vi "xml_get_target.vi"(3 "error in (no error)":errorcluster, 4 "XML Path":path=path "D:/Test Management/Farmer/XML/targets.xml", 5 "target name":string) -> (0 "error out":errorcluster, 1 "success?":bool, 2 "Data":T1)   [LabVIEW 2011]
uses:
  TargetData.ctl
  <vilib>/xml/Load XML File.vi
  <vilib>/xml/Close Reference(Node).vi
  <vilib>/xml/NI_XML.lvlib
  Program Files/National Instruments/LabVIEW 2011/resource/objmgr/DOMUserDefRef.rc
panel:
  in  "data type":T1
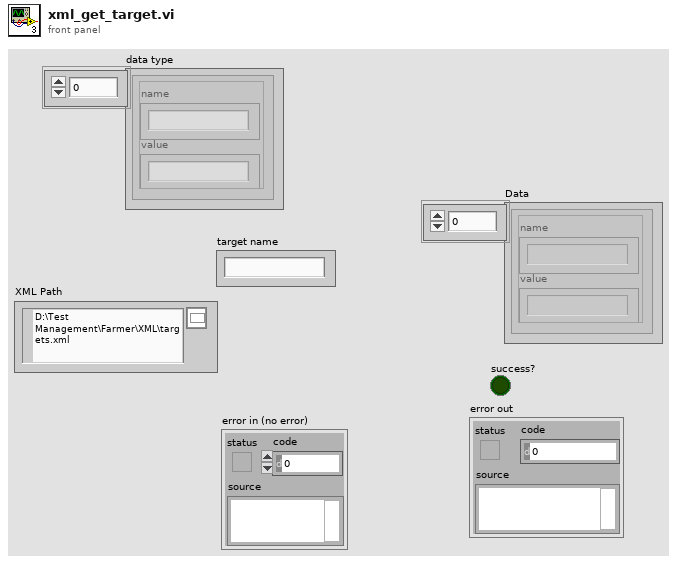
[diagram p1: front panel]
types:
  T1 = typedef "TargetData.ctl" = cluster{"name":string, "value":string}[]
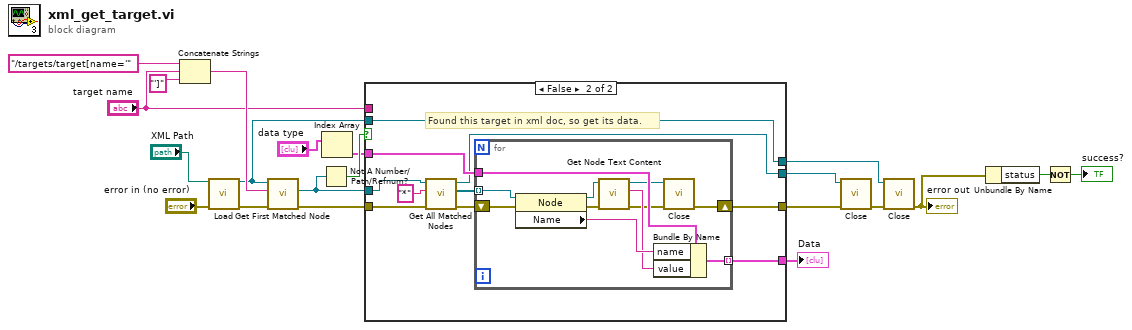
[diagram p0: block diagram]
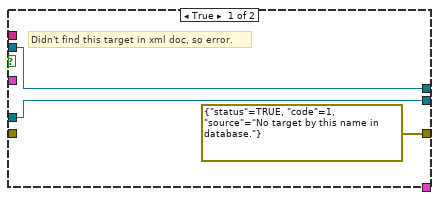
[diagram p2: hidden frame]
diagram:
  n1 = Concatenate Strings("/targets/target[name='", "target name", "']") -> (w19:string)
  n2 = call-poly <vilib>:"Load.vi"("path to XML document"="XML Path", "error in (no error)"="error in (no error)") -> ("DOM document out"=w6:refnum<k20>, "error out"=w18:errorcluster)  [unwired: 11 in, 1 out]
  n3 = call <vilib>:"Get First Matched Node.vi"("error in (no error)"=w18, "XPath expression"=w19, "node in"=w6) -> ("error out"=w17:errorcluster, "node result"=w14:refnum<k20>)  [unwired: 6 in, 1 out]
  n4 = Not A Number/Path/Refnum?(number/path/refnum=w14) -> (NaN/Path/Refnum?=w16:bool)
  n5 = Index Array(array="data type") -> (element=w3:cluster{"name":string, "value":string})  [unwired: 1 in]
  n6 = case shown="False" w16 {
    tunnel: w17 -> [_ w31]
    tunnel: [errorcluster {"status"=TRUE, "code"=1, "source"="No target by this name in database."} ("error out") w25] -> w8
    tunnel: w14 -> [w23 w33]
    tunnel: "target name" -> [_ _]
    tunnel: [w23 w27] -> w7
    tunnel: w6 -> [w22 w34]
    tunnel: [w22 w34] -> w5
    tunnel: w3 -> [_ w28]
    tunnel: [_ w26] -> w2
    frame True {
      # "Didn't find this target in xml doc, so error."
    }
    frame False {
      # "Found this target in xml doc, so get its data."
      n7 = call <vilib>:"Get All Matched Nodes.vi"("error in (no error)"=w31, "XPath expression"="*", "node in"=w33) -> ("error out"=w29:errorcluster, "node result array"=w30:refnum<k20>[], "node out"=w27:refnum<k20>)  [unwired: 6 in]
      n8 = for {
        tunnel: w30 -> [w45] mode=indexing
        shift-right: [w36] -> w25
        shift-left: w29 -> [w43]
        tunnel: w28 -> [w41]
        tunnel: [w40] -> w26 mode=indexing
        n9 = property class="Node"(reference=w45, error in=w43) -> (reference out=w44:refnum<k20>, error out=w42:errorcluster, "Name"=w39:string)
        n10 = call <vilib>:"Get Node Text Content.vi"("error in (no error)"=w42, "node in"=w44) -> ("error out"=w37:errorcluster, "node text"=w38:string, "node out"=w35:refnum<k20>)  [unwired: 7 in]
        n11 = Bundle By Name(cluster=w41, "name"=w39, "value"=w38) -> (w40:cluster{"name":string, "value":string})
        n12 = call-poly <vilib>:"Close.vi"("error in (no error)"=w37, "node"=w35) -> ("error out"=w36:errorcluster)  [unwired: 7 in]
      }
    }
  }
  "Data" <- w2
  n13 = call-poly <vilib>:"Close.vi"("error in (no error)"=w8, "node"=w7) -> ("error out"=w15:errorcluster)  [unwired: 7 in]
  n14 = call-poly <vilib>:"Close.vi"("error in (no error)"=w15, "node"=w5) -> ("error out"=w12:errorcluster)  [unwired: 7 in]
  "error out" <- w12
  n15 = Unbundle By Name(w12) -> ("status"=w11:bool)
  n16 = Not(x=w11) -> (.not. x?=→"success?":bool)
